vi "QueenBuffer.vi"(0 "名称":T1, 4 "目标队列输入":refnum<queue>, 10 "操作":T2) -> (15 "目标队列":refnum<queue>)   [LabVIEW 2019]
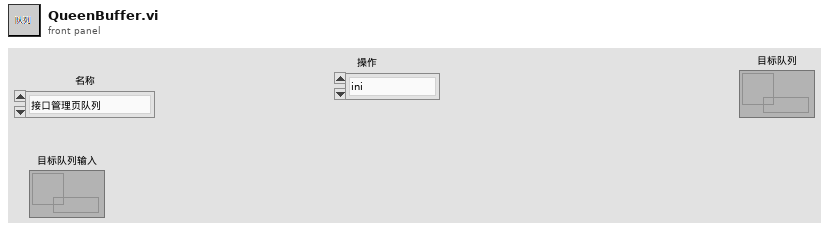
[diagram p1: front panel]
types:
  T1 = typedef "队列枚举1.ctl" = enum16{"接口管理页队列", "服务侦听页队列", "主页队列"}
  T2 = typedef "队列枚举.ctl" = enum16{"ini", "读", "写"}
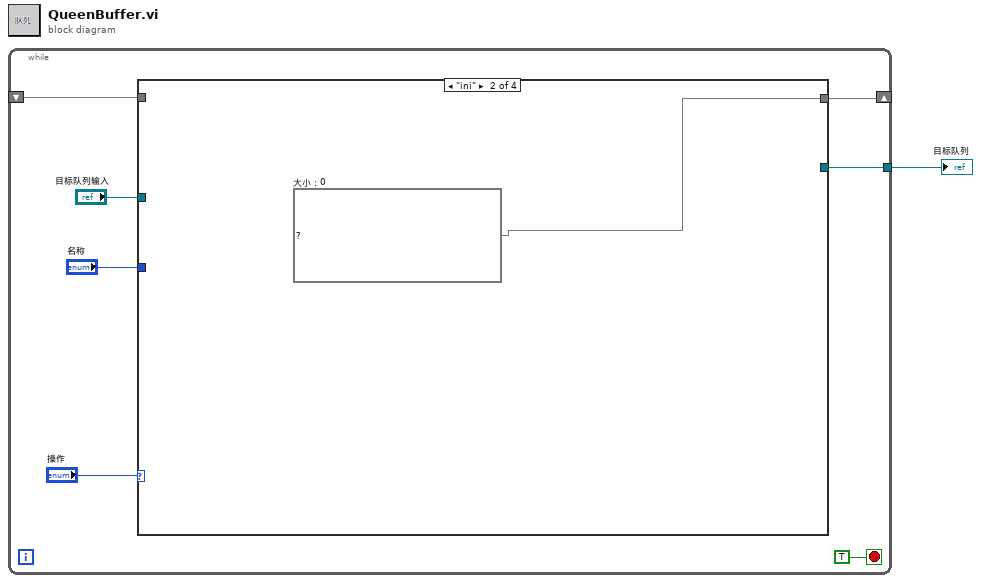
[diagram p0: block diagram]
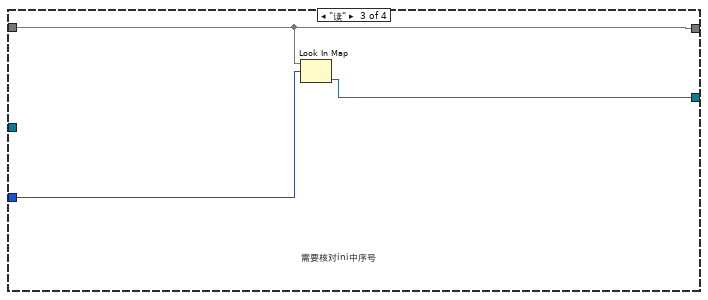
[diagram p3: hidden frame]
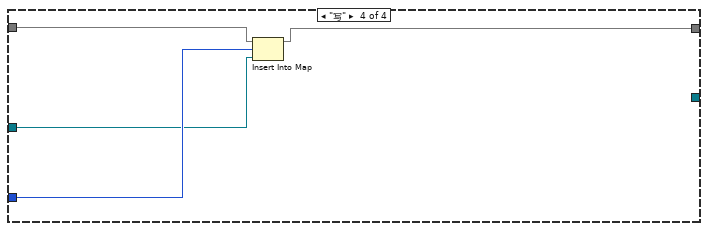
[diagram p4: hidden frame]
diagram:
  n1 = while {
    shift-right: [w6] -> _
    shift-left: _ -> [w5]
    tunnel: [w4] -> w1
    stop <- TRUE stop-if-true
    n2 = case shown="\"ini\"" "操作" {
      tunnel: [w9 w10 w13 w16] -> w6
      tunnel: w5 -> [w9 _ w13 w17]
      tunnel: [_ _ w11 _] -> w4
      tunnel: "名称" -> [_ _ w12 w15]
      tunnel: "目标队列输入" -> [_ _ _ w14]
      frame Default {
      }
      frame "ini" {
        w10 = map{T1, refnum<queue>} {}  # 大小：0
      }
      frame "读" {
        # "需要核对ini中序号"
        n3 = Look In Map(map=w13, key=w12) -> (value=w11:refnum<queue>)  [unwired: 1 in, 1 out]
      }
      frame "写" {
        n4 = Insert Into Map(map in=w17, key=w15, value=w14) -> (map out=w16:map{T1, refnum<queue>})  [unwired: 2 out]
      }
    }
  }
  "目标队列" <- w1
